vi "Store Current Measurment.vi"(8 "error in":errorcluster, 10 "Value":dbl, 11 "Measurement":T1) -> (0 "error out":errorcluster)   [LabVIEW 2016, in "Hall Effect Library.lvlib"]
uses:
  Hall Effect Library.lvlib
  Controls/Measurement.ctl
  Global Variables/Hall Effect Data.vi
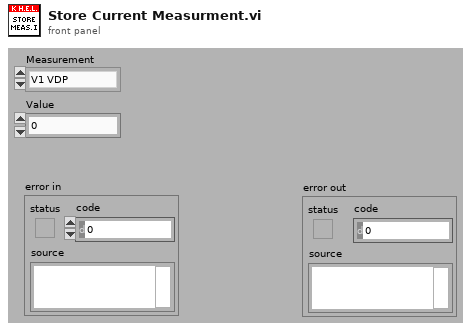
[diagram p1: front panel]
types:
  T1 = typedef "Hall Effect Library.lvlib/Measurement.ctl" = enum16{"V1 VDP", "V2 VDP", "V3 VDP", "V4 VDP", "V5 VDP", "V6 VDP", "V7 VDP", "V8 VDP", "V1 HE", "V2 HE", "V3 HE", "V4 HE", "V5 HE", "V6 HE", "V7 HE", "V8 HE", "V1 Res Bar", "V1 Hall Bar", "V1 Res 6-Cot", "V2 Res 6-Cot", "V3 Res 6-Cot", "V4 Res 6-Cot", "V1 Hall 6-Cot", "V2 Hall 6-Cot", "V3 Hall 6-Cot", "V4 Hall 6-Cot", "V5 Hall 6-Cot", "V6 Hall 6-Cot", "V7 Hall 6-Cot", "V8 Hall 6-Cot", "V1 Res 8-Cot", "V2 Res 8-Cot", "V3 Res 8-Cot", "V4 Res 8-Cot", "V1 Hall 8-Cot", "V2 Hall 8-Cot", "V3 Hall 8-Cot", "V4 Hall 8-Cot"}
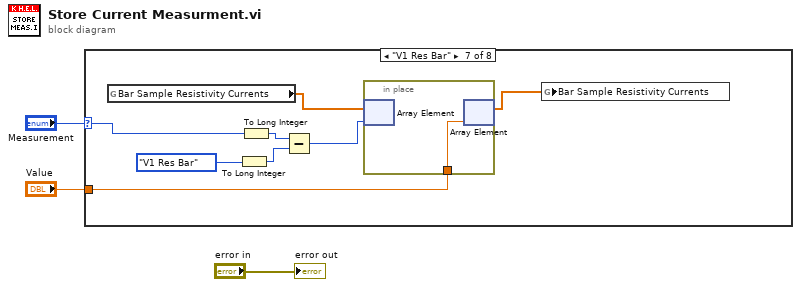
[diagram p0: block diagram]
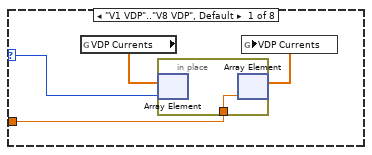
[diagram p2: hidden frame]
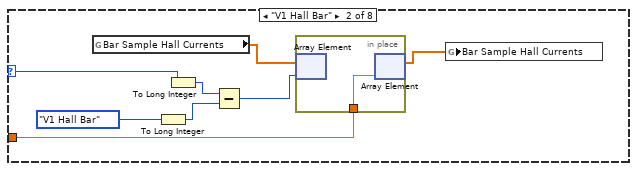
[diagram p3: hidden frame]
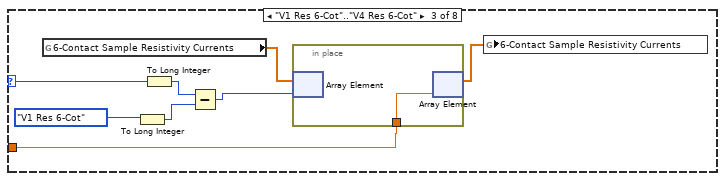
[diagram p4: hidden frame]
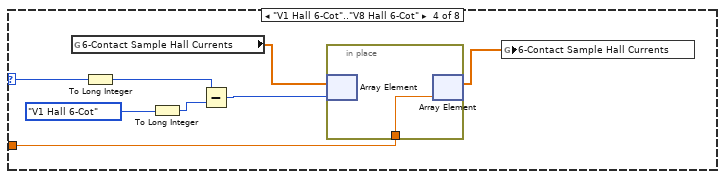
[diagram p5: hidden frame]
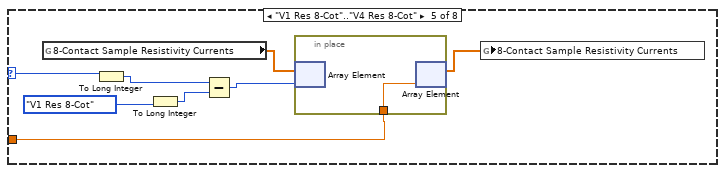
[diagram p6: hidden frame]
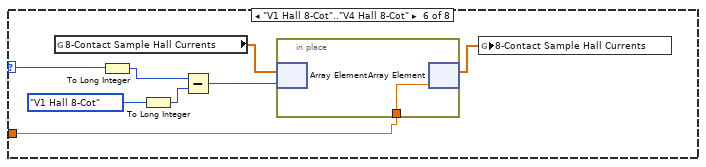
[diagram p7: hidden frame]
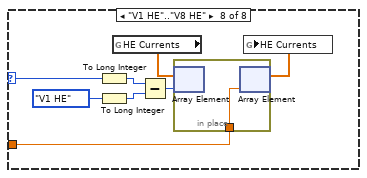
[diagram p8: hidden frame]
diagram:
  n1 = case shown="\"V1 Res Bar\"" "Measurement" {
    selector: "Measurement" -> [w6 w13 w25 w31 w40 w49 w58 w63]
    tunnel: "Value" -> [w5 w14 w22 w32 w41 w50 w61 w67]
    frame "V1 VDP".."V8 VDP", Default {
      n2 = global read "Hall Effect Data.vi" "VDP Currents"() -> (w7:dbl[])
      n3 = in-place {
        in-place-border: w5 -> [w8]
        n4 = in-place-array #1(w7, w6) -> ()  [unwired: 1 out]
        n5 = in-place-array #1(w8) -> (w4:dbl[])  [unwired: 1 out]
      }
      n6 = global write "Hall Effect Data.vi" "VDP Currents"(w4) -> ()
    }
    frame "V1 Hall Bar" {
      n7 = global read "Hall Effect Data.vi" "Bar Sample Hall Currents"() -> (w16:dbl[])
      n8 = To Long Integer(number=Measurement."V1 Hall Bar" ("y")) -> (32bit integer=w10:i32)
      n9 = To Long Integer(number=w13) -> (32bit integer=w11:i32)
      n10 = Subtract(x=w11, y=w10) -> (x-y=w9:i32)
      n11 = in-place {
        in-place-border: w14 -> [w17]
        n12 = in-place-array #2(w16, w9) -> ()  [unwired: 1 out]
        n13 = in-place-array #2(w17) -> (w15:dbl[])  [unwired: 1 out]
      }
      n14 = global write "Hall Effect Data.vi" "Bar Sample Hall Currents"(w15) -> ()
    }
    frame "V1 Res 6-Cot".."V4 Res 6-Cot" {
      n15 = global read "Hall Effect Data.vi" "6-Contact Sample Resistivity Currents"() -> (w24:dbl[])
      n16 = To Long Integer(number=Measurement."V1 Res 6-Cot" ("y")) -> (32bit integer=w19:i32)
      n17 = To Long Integer(number=w25) -> (32bit integer=w20:i32)
      n18 = Subtract(x=w20, y=w19) -> (x-y=w18:i32)
      n19 = in-place {
        in-place-border: w22 -> [w26]
        n20 = in-place-array #3(w24, w18) -> ()  [unwired: 1 out]
        n21 = in-place-array #3(w26) -> (w23:dbl[])  [unwired: 1 out]
      }
      n22 = global write "Hall Effect Data.vi" "6-Contact Sample Resistivity Currents"(w23) -> ()
    }
    frame "V1 Hall 6-Cot".."V8 Hall 6-Cot" {
      n23 = global read "Hall Effect Data.vi" "6-Contact Sample Hall Currents"() -> (w34:dbl[])
      n24 = To Long Integer(number=w31) -> (32bit integer=w29:i32)
      n25 = To Long Integer(number=Measurement."V1 Hall 6-Cot" ("y")) -> (32bit integer=w28:i32)
      n26 = Subtract(x=w29, y=w28) -> (x-y=w27:i32)
      n27 = in-place {
        in-place-border: w32 -> [w35]
        n28 = in-place-array #4(w34, w27) -> ()  [unwired: 1 out]
        n29 = in-place-array #4(w35) -> (w33:dbl[])  [unwired: 1 out]
      }
      n30 = global write "Hall Effect Data.vi" "6-Contact Sample Hall Currents"(w33) -> ()
    }
    frame "V1 Res 8-Cot".."V4 Res 8-Cot" {
      n31 = global read "Hall Effect Data.vi" "8-Contact Sample Resistivity Currents"() -> (w43:dbl[])
      n32 = To Long Integer(number=w40) -> (32bit integer=w38:i32)
      n33 = To Long Integer(number=Measurement."V1 Res 8-Cot" ("y")) -> (32bit integer=w37:i32)
      n34 = Subtract(x=w38, y=w37) -> (x-y=w36:i32)
      n35 = in-place {
        in-place-border: w41 -> [w44]
        n36 = in-place-array #5(w43, w36) -> ()  [unwired: 1 out]
        n37 = in-place-array #5(w44) -> (w42:dbl[])  [unwired: 1 out]
      }
      n38 = global write "Hall Effect Data.vi" "8-Contact Sample Resistivity Currents"(w42) -> ()
    }
    frame "V1 Hall 8-Cot".."V4 Hall 8-Cot" {
      n39 = global read "Hall Effect Data.vi" "8-Contact Sample Hall Currents"() -> (w52:dbl[])
      n40 = To Long Integer(number=w49) -> (32bit integer=w46:i32)
      n41 = To Long Integer(number=Measurement."V1 Hall 8-Cot" ("y")) -> (32bit integer=w47:i32)
      n42 = Subtract(x=w46, y=w47) -> (x-y=w45:i32)
      n43 = in-place {
        in-place-border: w50 -> [w53]
        n44 = in-place-array #6(w52, w45) -> ()  [unwired: 1 out]
        n45 = in-place-array #6(w53) -> (w51:dbl[])  [unwired: 1 out]
      }
      n46 = global write "Hall Effect Data.vi" "8-Contact Sample Hall Currents"(w51) -> ()
    }
    frame "V1 Res Bar" {
      n47 = global read "Hall Effect Data.vi" "Bar Sample Resistivity Currents"() -> (w60:dbl[])
      n48 = To Long Integer(number=Measurement."V1 Res Bar" ("y")) -> (32bit integer=w55:i32)
      n49 = To Long Integer(number=w58) -> (32bit integer=w56:i32)
      n50 = Subtract(x=w56, y=w55) -> (x-y=w54:i32)
      n51 = in-place "In Place Element Structure" {
        in-place-border: w61 -> [w62]
        n52 = in-place-array #7(w60, w54) -> ()  [unwired: 1 out]
        n53 = in-place-array #7(w62) -> (w59:dbl[])  [unwired: 1 out]
      }
      n54 = global write "Hall Effect Data.vi" "Bar Sample Resistivity Currents"(w59) -> ()
    }
    frame "V1 HE".."V8 HE" {
      n55 = To Long Integer(number=w63) -> (32bit integer=w66:i32)
      n56 = To Long Integer(number=Measurement."V1 HE" ("y")) -> (32bit integer=w65:i32)
      n57 = global read "Hall Effect Data.vi" "HE Currents"() -> (w70:dbl[])
      n58 = Subtract(x=w66, y=w65) -> (x-y=w68:i32)
      n59 = in-place {
        in-place-border: w67 -> [w71]
        n60 = in-place-array #8(w70, w68) -> ()  [unwired: 1 out]
        n61 = in-place-array #8(w71) -> (w69:dbl[])  [unwired: 1 out]
      }
      n62 = global write "Hall Effect Data.vi" "HE Currents"(w69) -> ()
    }
  }
  "error out" <- "error in"
